vi "TL find arbiter max value B.vi"(0 "ACT array":dbl[](array[numeric]), 1 "error in":errorcluster) -> (2 "Peak Heading":dbl, 3 "Max value":dbl, 4 "error out":errorcluster)   [LabVIEW 2014]
doc: "This is the arbiter peak detector for the SSB midbrain. It finds the max value closest to a heading of 0/360 degrees."
panel:
  out "Positive Max?":bool
  out "Peak index":dbl
  out "Arbiter array Graph":cluster{dbl, dbl, "ACT array":dbl[]}(graph)
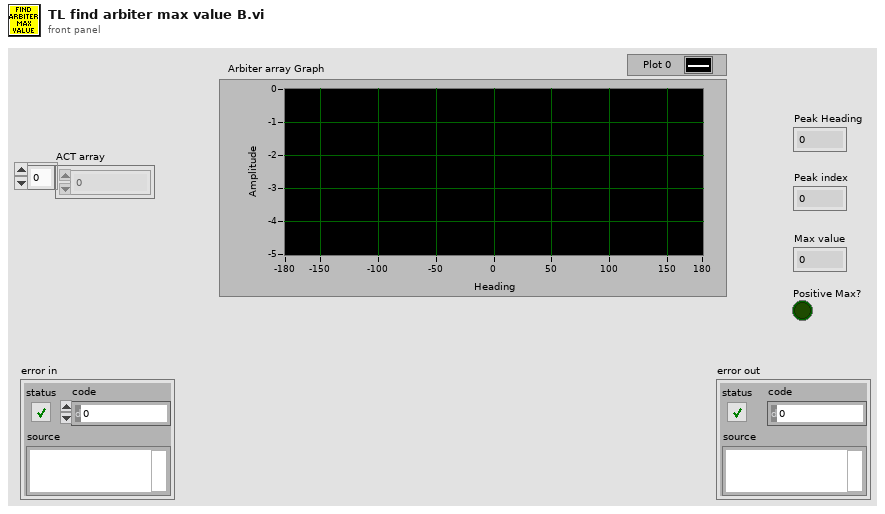
[diagram p1: front panel]
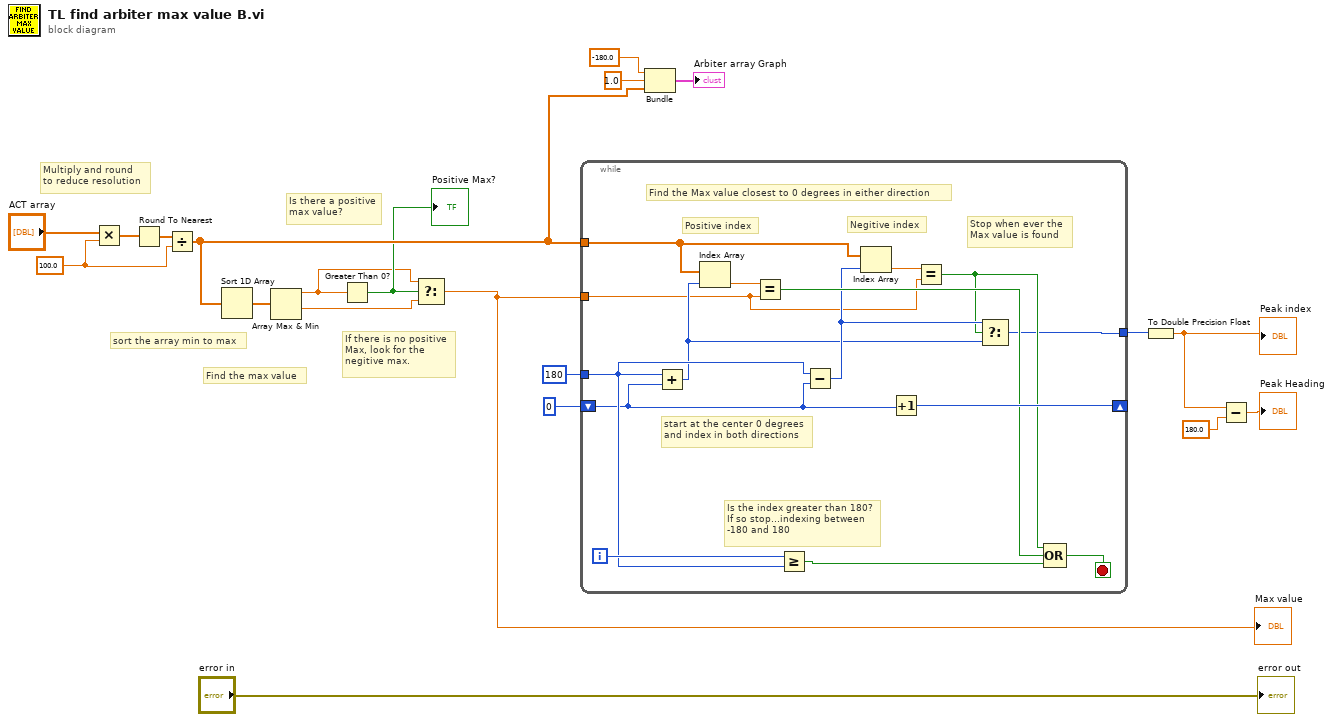
[diagram p0: block diagram]
diagram:
  w9 = 100.0
  # "If there is no positive\nMax, look for the \nnegitive max."
  # "Is there a positive\nmax value?"
  # "Multiply and round\nto reduce resolution"
  # "Find the max value"
  # "sort the array min to max"
  n1 = Multiply(x="ACT array", y=w9) -> (x*y=w13:dbl[])
  n2 = Round To Nearest(number=w13) -> (nearest integer value=w10:dbl[])
  n3 = Divide(x=w10, y=w9) -> (x/y=w8:dbl[])
  n4 = Sort 1D Array(array=w8) -> (sorted array=w11:dbl[])
  n5 = Array Max & Min(array=w11) -> (max value=w3:dbl, min value=w1:dbl)  [unwired: 2 out]
  n6 = Greater Than 0?(x=w3) -> (x > 0?=w4:bool)
  "Positive Max?" <- w4
  n7 = Select(t=w3, s=w4, f=w1) -> (s? t:f=w2:dbl)
  "Max value" <- w2
  n8 = while {
    tunnel: w2 -> [w23]
    tunnel: w8 -> [w22]
    shift-right: [w35] -> _
    shift-left: 0 -> [w29]
    tunnel: [w24] -> w14
    tunnel: 180 -> [w30]
    i -> [w34]
    stop <- w31 stop-if-true
    # "Stop when ever the\nMax value is found"
    # "Negitive index"
    # "Positive index"
    # "Is the index greater than 180?\nIf so stop...indexing between\n-180 and 180"
    # "start at the center 0 degrees\nand index in both directions"
    # "Find the Max value closest to 0 degrees in either direction"
    n9 = Add(x=w30, y=w29) -> (x+y=w25:i32)
    n10 = Index Array(array=w22, index=w25) -> (element=w21:dbl)
    n11 = Equal?(x=w21, y=w23) -> (x = y?=w32:bool)
    n12 = Greater Or Equal?(x=w34, y=w30) -> (x >= y?=w33:bool)
    n13 = Subtract(x=w30, y=w29) -> (x-y=w27:i32)
    n14 = Index Array(array=w22, index=w27) -> (element=w28:dbl)
    n15 = Increment(x=w29) -> (x+1=w35:i32)
    n16 = Equal?(x=w28, y=w23) -> (x = y?=w26:bool)
    n17 = Select(t=w27, s=w26, f=w25) -> (s? t:f=w24:i32)
    n18 = Compound Arithmetic op=OR(w26, w32, w33) -> (w31:bool)
  }
  n19 = Bundle(-180.0, 1.0, w8) -> (→"Arbiter array Graph":cluster{dbl, dbl, dbl[]})  [unwired: 1 in]
  n20 = To Double Precision Float(number=w14) -> (double precision float=w5:dbl)
  "Peak index" <- w5
  n21 = Subtract(x=w5, y=180.0) -> (x-y=→"Peak Heading":dbl)
  "error out" <- "error in"
